vi "HighFrameRateRecording - DX cameras 2.vi"() -> ()   [LabVIEW 2014]
doc: "The LL Ring VI acquires images continuously and displays them in an image control using the low-level acquisition VIs. A ring initiates a continuous high-speed acquisition to multiple buffers and is appropriate for high-speed applications that perform processing on every image. Multiple buffers are useful when processing times vary depending on other applications and processing results .\n\nIMAQ Init initializes the device. IMAQ Configure List configures the buffer list with multiple buffers. IMAQ Create creates the image buffers. Call IMAQ Configure Buffer once for each buffer in the buffer list. IMAQ Start starts the acquisition, and IMAQ Extract Buffer ensures that the current image is not overwritten. An image control displays the image on the front panel. After exiting the loop, IMAQ Extract Buffer releases the last extracted buffer. IMAQ Close releases resources associated with the acquisition, and IMAQ Dispose frees the image buffer."
uses:
  <vilib>/vision/Avi.llb/IMAQ AVI2 Refnum.ctl
  <vilib>/userdefined/High Color/IMAQdx.ctl
  <vilib>/vision/driver/IMAQdx.llb/IMAQdx Acquisition Mode.ctl
  <vilib>/vision/driver/IMAQdx.llb/IMAQdx Buffer Number Mode.ctl
  <vilib>/vision/Avi.llb/IMAQ AVI2 Codec Path.ctl
  <vilib>/vision/driver/NI_Vision_Acquisition_Software.lvlib
  <vilib>/vision/NI_Vision_Development_Module.lvlib
panel:
  out "Buffer Number Out":u32=1403
  out "Frame Number":u32=1403
  out "Frame Rate Graph":dbl(graph)=30.03875968992248
  out "FPS":dbl=82.41758241758242 format="%#.1f"
  in  "Camera Selection DX":T1="cam3"
  out "AVI Refnum":T2
  out "Video recording":bool
  in  "Record?":bool
  in  "codec index":i32=5
  out "codec":string="Y800 Uncompressed Grey Scale (NI Vision)"
  in  "AVI File Path":path=path "E:/Video/gravity/1/30fps.avi"
  out "Processed Frames/s":dbl=30.03875968992248 format="%#.1g"
  in  "Stop":bool
  out "Saved Frames":i32
  out "Image":T3(plugin-control)
  # "ToDo:\n - add JSON output\n - andd indicator of _s# number"
  # "1.  Initialisation"
  # "Codec should be:\n\"Y800 Uncompressed Grey Scale\""
  # "Naming convention:\n - use the name above and add _s#.avi for videos\n - specs for saved videos is specified in name.json"
  # "2.  Recording"
  # "y"
  # "Record"
  # "x"
  # "Just Observe"
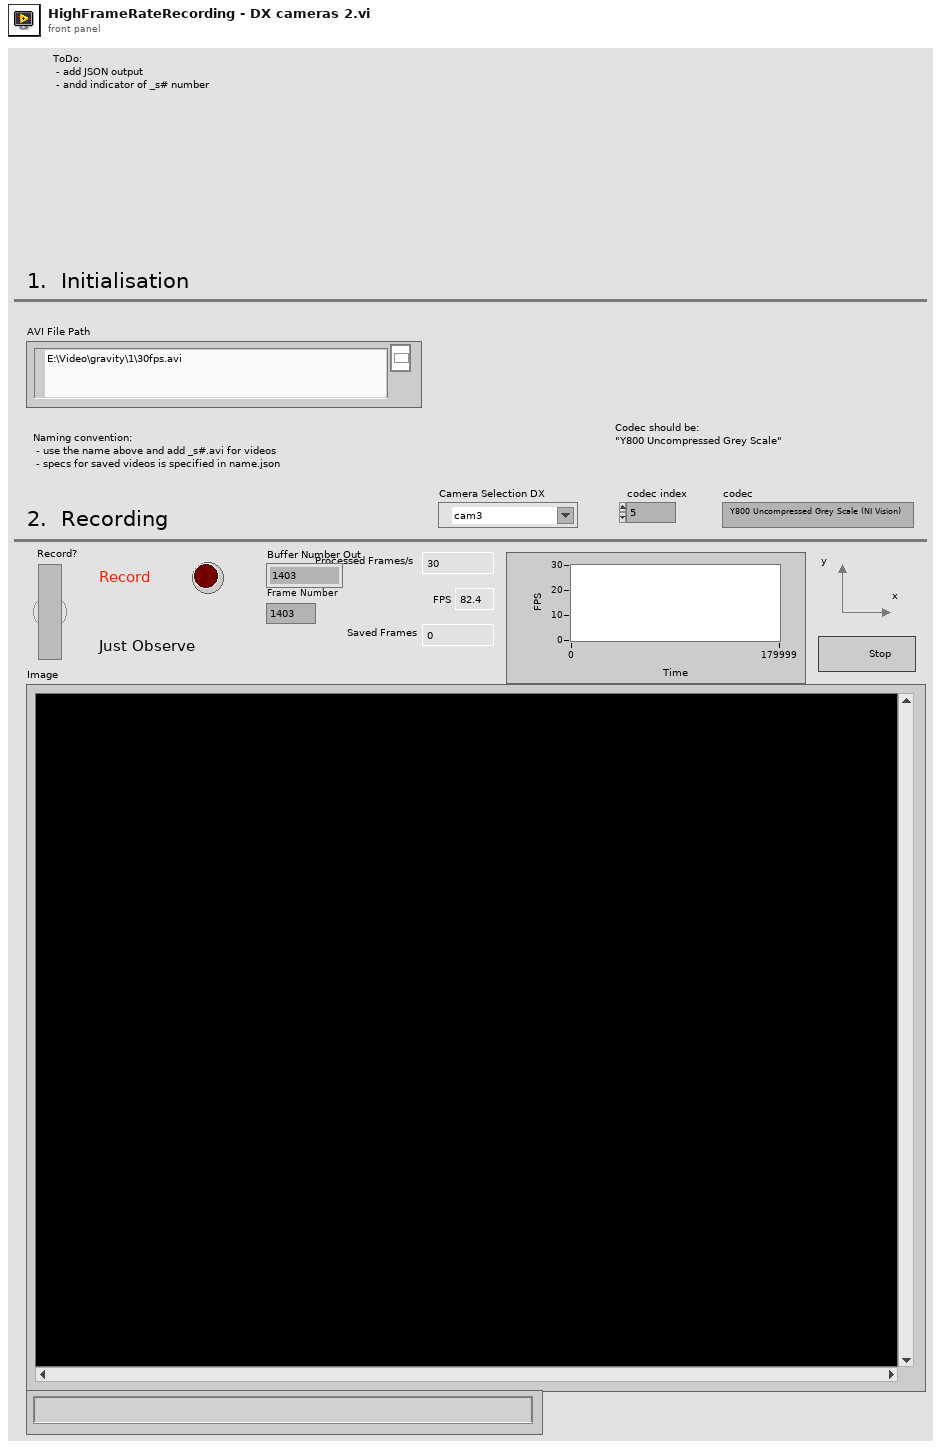
[diagram p1: front panel]
types:
  T1 = typedef "IMAQdx.ctl" = refnum<k21>
  T2 = typedef "IMAQ AVI2 Refnum.ctl" = refnum<k20>
  T3 = typedef "IMAQ Image.ctl" = refnum<image>
  T4 = typedef "Image Type" = u32
  T5 = typedef "NI_Vision_Acquisition_Software.lvlib/IMAQdx Acquisition Mode.ctl" = enum32{"One Shot", "Continuous"}
  T6 = typedef "IMAQ AVI2 Codec Path.ctl" = u32
  T7 = typedef "NI_Vision_Acquisition_Software.lvlib/IMAQdx Buffer Number Mode.ctl" = enum32{"Next", "Last", "Buffer Number", "Every", "Last New"}
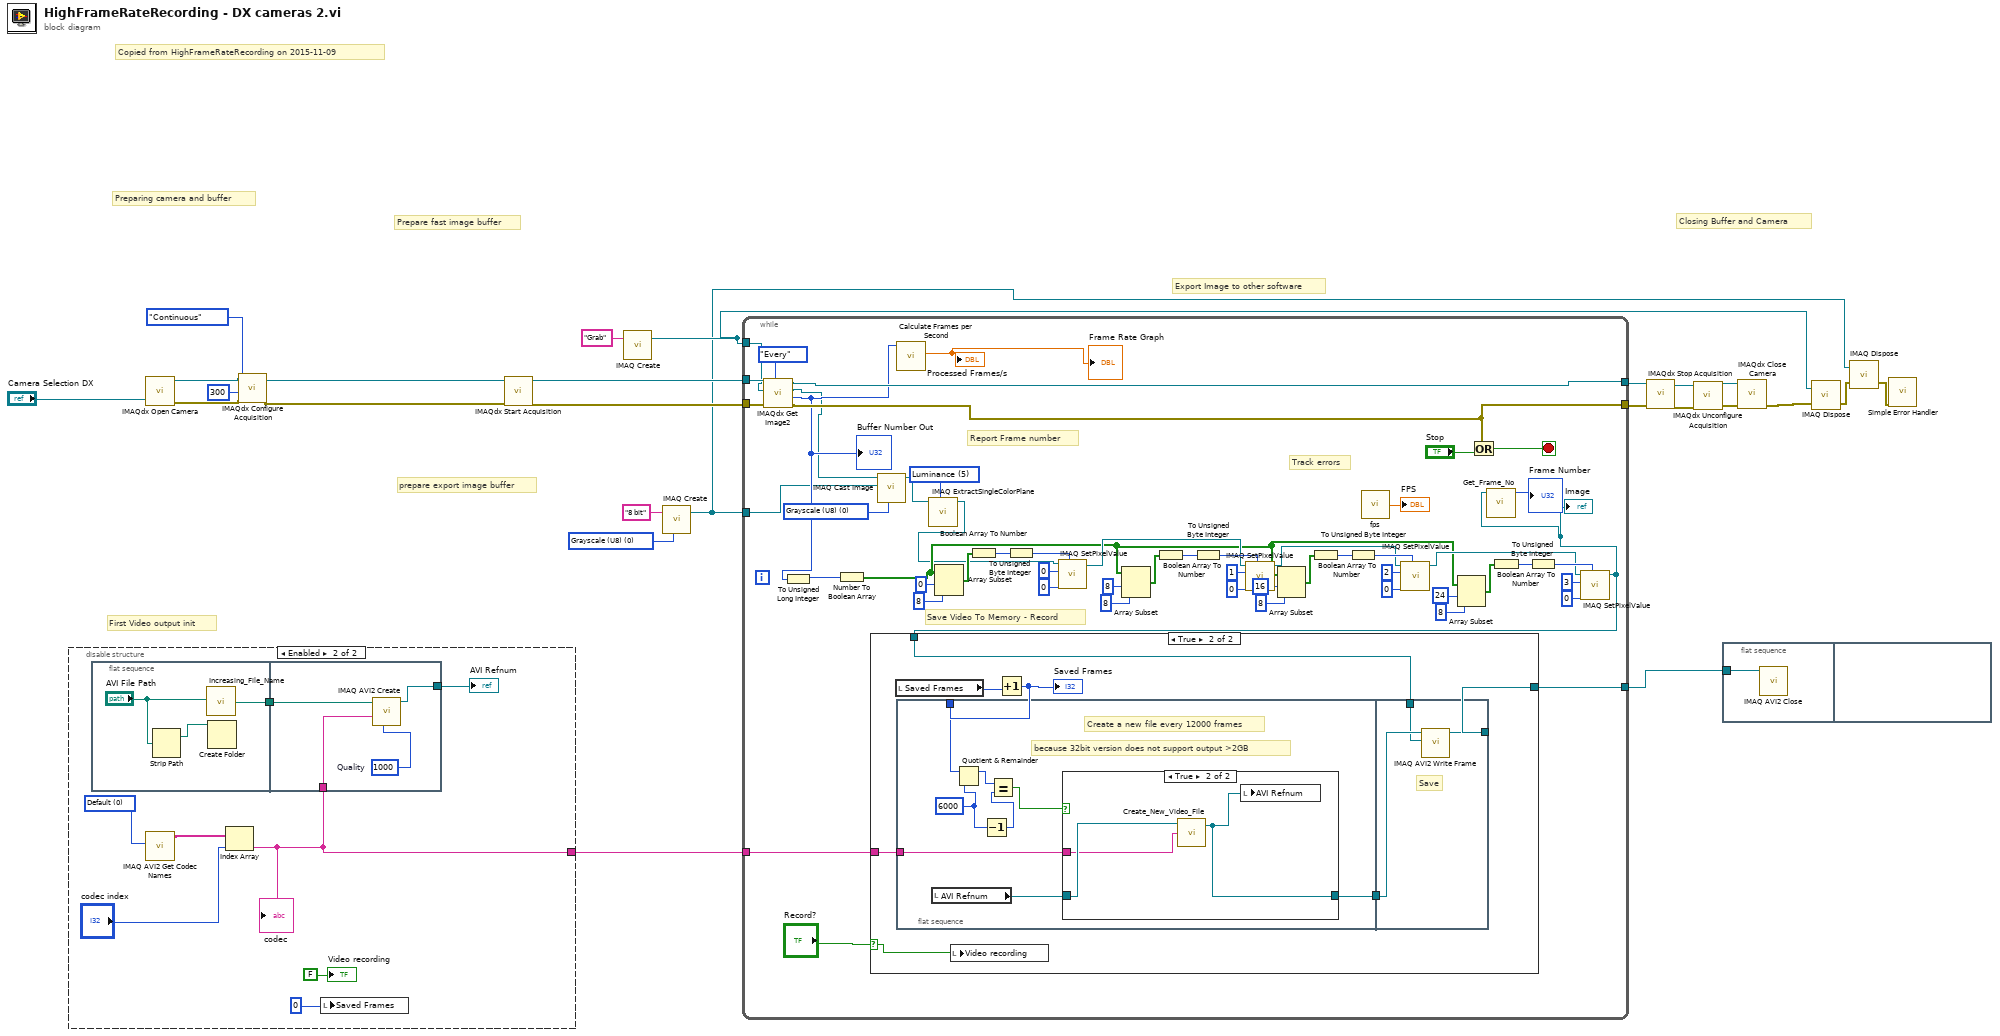
[diagram p0: block diagram]
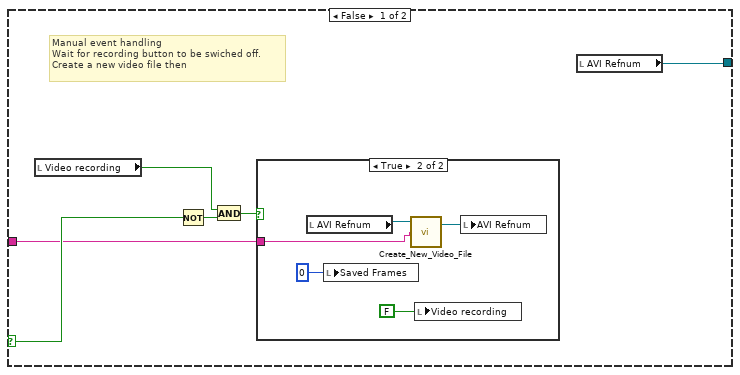
[diagram p3: hidden frame]
diagram:
  w1 = T4 0 items=["Grayscale (U8)", "Grayscale (I16)", "Grayscale (SGL)", "Complex (CSG)", "RGB (U32)", "HSL (U32)", "RGB (U64)", "Grayscale (U16)"] ("Image Type")
  # "Copied from HighFrameRateRecording on 2015-11-09"
  # "Export Image to other software"
  # "prepare export image buffer"
  # "Prepare fast image buffer"
  # "First Video output init"
  # "Closing Buffer and Camera"
  # "Preparing camera and buffer"
  n1 = disable-structure shown="Enabled" {
    disable-tunnel: [_ w26] -> w24
    frame Disabled {
    }
    frame Enabled {
      w33 = T6 0 items=["Default", "System", "Built in Vision"] ("Codec Source")
      n2 = flat-sequence {
        tunnel: [w36] -> w28
        tunnel: w28 -> [w38]
        tunnel: [w39] -> w27
        tunnel: w26 -> [w37]
        frame #0 {
          n3 = Strip Path(path="AVI File Path") -> (stripped path=w35:path)  [unwired: 1 out]
          n4 = call "Increasing_File_Name.vi"("Base AVI  path"="AVI File Path") -> ("Final AVI path"=w36:path)
          n5 = Create Folder(path (use dialog)=w35) -> ()  [unwired: 2 in, 3 out]
        }
        frame #1 {
          w40 = 1000  # Quality
          n6 = call "IMAQ AVI2 Create"("Quality"=w40, "Codec"=w37, "AVI Path"=w38) -> ("AVI Refnum"=w39:T2)  [unwired: 7 in, 1 out]
        }
      }
      n7 = call "IMAQ AVI2 Get Codec Names"("Codec Source"=w33) -> ("Codec Names"=w32:string[])  [unwired: 9 in, 1 out]
      n8 = Index Array(array=w32, index="codec index") -> (element=w26:string)
      "codec" <- w26
      n9 = local write "Saved Frames"(0 ("Saved Frames")) -> ()
      "AVI Refnum" <- w27
      "Video recording" <- FALSE ("Video recording")
    }
  }
  n10 = call <vilib>:"IMAQdx Open Camera.vi"("Session In"="Camera Selection DX") -> ("error out"=w19:errorcluster, "Session Out"=w18:T1)  [unwired: 9 in]
  n11 = call <vilib>:"IMAQdx Configure Acquisition.vi"("error in"=w19, "Number of Buffers"=u32 300, "Continuous?"=IMAQdx_Acquisition_Mode."Continuous", "Session In"=w18) -> ("error out"=w12:errorcluster, "Session Out"=w13:T1)  [unwired: 6 in]
  n12 = call <vilib>:"IMAQdx Start Acquisition.vi"("error in"=w12, "Session In"=w13) -> ("error out"=w14:errorcluster, "Session Out"=w15:T1)  [unwired: 8 in]
  n13 = call "IMAQ Create"("Image Name"="Grab") -> ("New Image"=w20:T3)  [unwired: 3 in, 2 out]
  n14 = call "IMAQ Create"("Image Name"="8 bit", "Image Type"=w1) -> ("New Image"=w2:T3)  [unwired: 2 in, 2 out]
  n15 = while {
    tunnel: [w84] -> w7
    tunnel: [w85] -> w6
    tunnel: [w92] -> w25
    tunnel: w24 -> [w91]
    tunnel: w15 -> [w88]
    tunnel: w14 -> [w86]
    tunnel: w20 -> [w87]
    tunnel: w2 -> [w45]
    stop <- w95 stop-if-true
    w41 = 5 items=["Red", "Green", "Blue", "Hue", "Saturation", "Luminance", "Value", "Intensity"] ("Color Plane")
    w47 = T4 0 items=["Grayscale (U8)", "Grayscale (I16)", "Grayscale (SGL)", "Complex (CSG)", "RGB (U32)", "HSL (U32)", "RGB (U64)", "Grayscale (U16)"] ("Image Type")
    # "Track errors"
    # "Report Frame number"
    # "Save Video To Memory - Record"
    n16 = call <vilib>:"IMAQdx Get Image2.vi"("Buffer Number Mode (Next)"=IMAQdx_Buffer_Number_Mode."Every", "error in"=w86, "Image In"=w87, "Session In"=w88) -> ("error out"=w85:errorcluster, "Buffer Number Out"=w48:u32, "Image Out"=w46:T3, "Session Out"=w84:T1)  [unwired: 4 in]
    "Buffer Number Out" <- w48
    n17 = To Unsigned Long Integer(number=w48) -> (unsigned 32bit integer=w82:u32)
    n18 = Number To Boolean Array(number=w82) -> (Boolean array=w50:bool[])
    n19 = call "IMAQ Cast Image"("Image Type"=w47, "Image Dst"=w45, "Image Src"=w46) -> ("Image Dst Out"=w43:T3)  [unwired: 7 in, 1 out]
    n20 = call <vilib>:"Calculate Frames per Second.vi"("Buffer Number"=w48) -> ("Processed Frames/s"=→"Processed Frames/s" →"Frame Rate Graph":dbl)  [unwired: 8 in, 2 out]
    n21 = call "IMAQ ExtractSingleColorPlane"("Color Plane"=w41, "Image Src"=w43) -> ("Image Dst Out"=w42:T3)  [unwired: 8 in, 1 out]
    n22 = Array Subset(array=w50, index=0, length=8) -> (w81:bool[])
    n23 = Boolean Array To Number(Boolean array=w81) -> (number=w80:u32)
    n24 = To Unsigned Byte Integer(number=w80) -> (unsigned 8bit integer=w79:u8)
    n25 = call "IMAQ SetPixelValue"("Pixel Value"=w79, "Y Coordinate"=0, "X Coordinate"=0, "Image"=w42) -> ("Image Out"=w60:T3)  [unwired: 6 in, 1 out]
    n26 = Array Subset(array=w50, index=8, length=8) -> (w74:bool[])
    n27 = Boolean Array To Number(Boolean array=w74) -> (number=w73:u32)
    n28 = To Unsigned Byte Integer(number=w73) -> (unsigned 8bit integer=w72:u8)
    n29 = call "IMAQ SetPixelValue"("Pixel Value"=w72, "Y Coordinate"=0, "X Coordinate"=1, "Image"=w60) -> ("Image Out"=w59:T3)  [unwired: 6 in, 1 out]
    n30 = Array Subset(array=w50, index=16, length=8) -> (w67:bool[])
    n31 = Boolean Array To Number(Boolean array=w67) -> (number=w66:u32)
    n32 = To Unsigned Byte Integer(number=w66) -> (unsigned 8bit integer=w65:u8)
    n33 = call "fps.vi"() -> ("FPS"=→"FPS":dbl)  [unwired: 1 in]
    n34 = call "IMAQ SetPixelValue"("Pixel Value"=w65, "Y Coordinate"=0, "X Coordinate"=2, "Image"=w59) -> ("Image Out"=w51:T3)  [unwired: 6 in, 1 out]
    n35 = Array Subset(array=w50, index=24, length=8) -> (w58:bool[])
    n36 = Or(x=w85, y="Stop") -> (x .or. y?=w95:bool)
    n37 = Boolean Array To Number(Boolean array=w58) -> (number=w57:u32)
    n38 = To Unsigned Byte Integer(number=w57) -> (unsigned 8bit integer=w56:u8)
    n39 = call "IMAQ SetPixelValue"("Pixel Value"=w56, "Y Coordinate"=0, "X Coordinate"=3, "Image"=w51) -> ("Image Out"=w44:T3)  [unwired: 6 in, 1 out]
    "Image" <- w44
    n40 = case shown="True" "Record?" {
      selector: "Record?" -> [w98 w108]
      tunnel: [w101 w111] -> w92
      tunnel: w44 -> [_ w109]
      tunnel: w91 -> [w96 w107]
      frame False {
        # "Manual event handling\nWait for recording button to be swiched off.\nCreate a new video file then"
        n41 = local read "Video recording"() -> (w97:bool)
        n42 = Not(x=w98) -> (.not. x?=w99:bool)
        n43 = And(x=w97, y=w99) -> (x .and. y?=w100:bool)
        n44 = case shown="True" w100 {
          tunnel: w96 -> [_ w102]
          frame False {
          }
          frame True {
            n45 = local read "AVI Refnum"() -> (w105:T2)
            n46 = local write "Saved Frames"(0 ("Saved Frames")) -> ()
            n47 = call "Create_New_Video_File.vi"("Codec"=w102, "AVI Refnum IN"=w105) -> ("AVI Refnum OUT"=w106:T2)  [unwired: 1 in, 1 out]
            n48 = local write "Video recording"(FALSE ("Video recording")) -> ()
            n49 = local write "AVI Refnum"(w106) -> ()
          }
        }
        n50 = local read "AVI Refnum"() -> (w101:T2)
      }
      frame True {
        n51 = local read "Saved Frames"() -> (w113:i32)
        n52 = flat-sequence {
          tunnel: w112 -> [w118]
          tunnel: [w115] -> w110
          tunnel: w107 -> [w114]
          tunnel: [w128] -> w111
          tunnel: w110 -> [w127]
          tunnel: w109 -> [w126]
          frame #0 {
            w120 = 6000 ("y")
            # "because 32bit version does not support output >2GB"
            # "Create a new file every 12000 frames"
            n53 = local read "AVI Refnum"() -> (w116:T2)
            n54 = Quotient & Remainder(x=w118, y=w120) -> (x-y*floor(x/y)=w121:i32)  [unwired: 1 out]
            n55 = Decrement(x=w120) -> (x-1=w119:i32)
            n56 = Equal?(x=w121, y=w119) -> (x = y?=w117:bool)
            n57 = case shown="True" w117 {
              tunnel: w116 -> [w122 w125]
              tunnel: [w122 w124] -> w115
              tunnel: w114 -> [_ w123]
              frame False {
              }
              frame True {
                n58 = call "Create_New_Video_File.vi"("Codec"=w123, "AVI Refnum IN"=w125) -> ("AVI Refnum OUT"=w124:T2)  [unwired: 1 in, 1 out]
                n59 = local write "AVI Refnum"(w124) -> ()
              }
            }
          }
          frame #1 {
            # "Save"
            n60 = call "IMAQ AVI2 Write Frame"("Image"=w126, "AVI Refnum"=w127) -> ("AVI Refnum (duplicate)"=w128:T2)  [unwired: 7 in, 2 out]
          }
        }
        n61 = local write "Video recording"(w108) -> ()
        n62 = Increment(x=w113) -> (x+1=w112:i32)
        "Saved Frames" <- w112
      }
    }
    n63 = call "Get_Frame_No.vi"("Image In"=w44) -> ("Frame Number"=→"Frame Number":u32)  [unwired: 10 in]
  }
  n64 = call <vilib>:"IMAQdx Stop Acquisition.vi"("error in"=w6, "Session In"=w7) -> ("error out"=w8:errorcluster, "Session Out"=w9:T1)  [unwired: 8 in]
  n65 = call <vilib>:"IMAQdx Unconfigure Acquisition.vi"("error in"=w8, "Session In"=w9) -> ("error out"=w10:errorcluster, "Session Out"=w11:T1)  [unwired: 8 out]
  n66 = flat-sequence {
    tunnel: w25 -> [w129]
    frame #0 {
      n67 = call "IMAQ AVI2 Close"("AVI Refnum"=w129) -> ()  [unwired: 10 in, 1 out]
    }
    frame #1 {
    }
  }
  n68 = call <vilib>:"IMAQdx Close Camera.vi"("error in"=w10, "Session In"=w11) -> ("error out"=w22:errorcluster)  [unwired: 9 in]
  n69 = call "IMAQ Dispose"("Image"=w20, "error in (no error)"=w22) -> ("error out"=w4:errorcluster)  [unwired: 1 in, 3 out]
  n70 = call "IMAQ Dispose"("Image"=w2, "error in (no error)"=w4) -> ("error out"=w3:errorcluster)  [unwired: 1 in, 3 out]
  n71 = call <vilib>:"Simple Error Handler.vi"("error in (no error)"=w3) -> ()  [unwired: 1 in, 8 out]
